vi "Modify Element.vi"(8 "g":dbl, 9 "f":dbl, 10 "index":i32, 11 "Priority Queue in":refnum<class "NI_Robotics_Priority Queue.lvclass">) -> (3 "Priority Queue out":refnum<class "NI_Robotics_Priority Queue.lvclass">)   [LabVIEW 2017, in "NI_Robotics_Priority Queue.lvclass"]
uses:
  <vilib>/robotics/Navigation/shared/Priority Queue/NI_Robotics_Priority Queue.lvclass
  <vilib>/robotics/Navigation/shared/Priority Queue/NI_Robotics_Priority Queue.lvclass/NI_Robotics_Priority Queue.ctl
  <vilib>/robotics/Navigation/shared/Priority Queue/Open List Element.ctl
  <vilib>/robotics/Navigation/shared/MapNode/AbstractMapNode/NI_Robotics_AbstractMapNode.lvclass
panel:
  # "Sets the f and g values of the element specified at index"
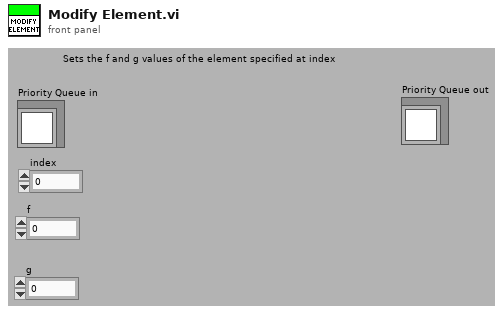
[diagram p1: front panel]
types:
  T1 = typedef "NI_Robotics_Priority Queue.lvclass/Open List Element.ctl" = cluster{"f":dbl, "g":dbl, "node Ref":refnum<data-value>}
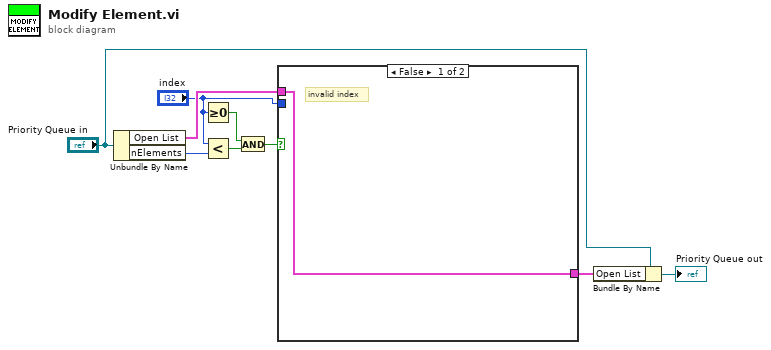
[diagram p0: block diagram]
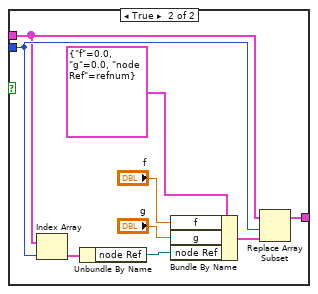
[diagram p2: hidden frame]
diagram:
  n1 = Unbundle By Name("Priority Queue in") -> ("Open List"=w6:T1[], "nElements"=w3:i32)
  n2 = Greater Or Equal To 0?(x="index") -> (x >= 0?=w5:bool)
  n3 = Less?(x="index", y=w3) -> (x < y?=w2:bool)
  n4 = And(x=w5, y=w2) -> (x .and. y?=w1:bool)
  n5 = case shown="False" w1 {
    tunnel: [w10 w15] -> w9
    tunnel: "index" -> [_ w14]
    tunnel: w6 -> [w10 w13]
    frame False {
      # "invalid index"
    }
    frame True {
      n6 = Index Array(array=w13, index=w14) -> (element=w12:T1)
      n7 = Unbundle By Name(w12) -> ("node Ref"=w11:refnum<data-value>)
      n8 = Bundle By Name(cluster=T1 {"f"=0.0, "g"=0.0, "node Ref"=refnum} ("new element/subarray"), "f"="f", "g"="g", "node Ref"=w11) -> (w16:T1)
      n9 = Replace Array Subset(array=w13, new element=w16, index=w14) -> (w15:T1[])
    }
  }
  n10 = Bundle By Name(cluster="Priority Queue in", "Open List"=w9) -> (→"Priority Queue out":refnum<class "NI_Robotics_Priority Queue.lvclass">)
